vi "String to I64.vi"(8 "error in":errorcluster, 11 "Integer String":string) -> (0 "error out":errorcluster, 3 "I64":i64)   [LabVIEW 2020, in "CANopen.lvlib"]
doc: "Converts the string representation of a number in a specified base to an equivalent 32-bit signed integer."
uses:
  CANopen.lvlib
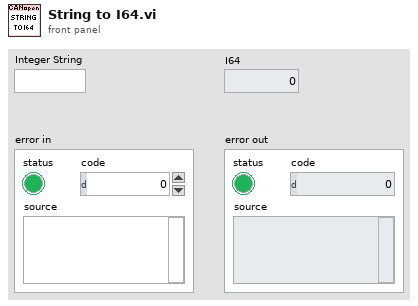
[diagram p1: front panel]
types:
  T1 = enum16{"U8", "U16", "U32", "I8", "I16", "I32", "I64", "U64"}
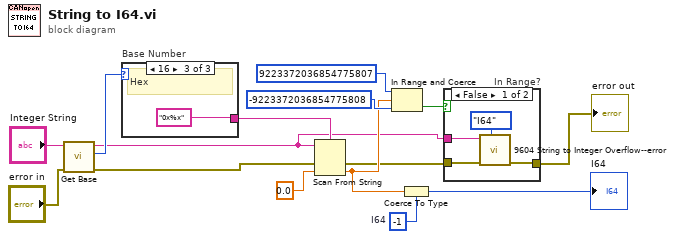
[diagram p0: block diagram]
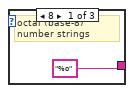
[diagram p3: hidden frame]
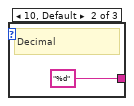
[diagram p4: hidden frame]
diagram:
  w2 = i64 -1  # I64
  n1 = call "Get Base.vi"("error in"="error in", "Default Value"="Integer String") -> ("error out"=w10:errorcluster, "Number Base"=w14:u8, "Default Value (dup)"=w1:string)  [unwired: 7 in]
  n2 = case "Base Number" shown="16" w14 {
    tunnel: ["%o" ("format string") "%d" ("format string") "0x%x" ("format string")] -> w12
    frame 8 {
      # "octal (base-8) number strings"
    }
    frame 10, Default {
      # "Decimal"
    }
    frame 16 {
      # "Hex"
    }
  }
  n3 = Scan From String(format string=w12, input string=w1, error in=w10, default 1=0.0 ("I32")) -> (error out=w6:errorcluster, output 1=w7:dbl)  [unwired: 1 in, 2 out]
  n4 = In Range and Coerce(upper limit=i64 9223372036854775807, x=w7, lower limit=i64 -9223372036854775808) -> (In Range?=w4:bool)  [unwired: 1 out]
  n5 = Coerce To Type(0:w7, 1:w2) -> (2:→"I64":i64)
  n6 = case "In Range?" shown="False" w4 {
    tunnel: w6 -> [w22 w23]
    tunnel: [w21 w23] -> w5
    tunnel: w1 -> [w20 _]
    frame False {
      n7 = call "9604 String to Integer Overflow--error.vi"("Type"=T1."I64", "error in"=w22, "Integer String"=w20) -> ("error out"=w21:errorcluster)  [unwired: 8 in]
    }
    frame True {
    }
  }
  "error out" <- w5
